vi "accel adjusted with gravity into ms2 (SubVI).vi"(10 "Array in":dbl[](array[numeric]), 11 "Array out":dbl[](array[numeric])) -> (3 "Array out":dbl[](array[numeric]))   [LabVIEW 2011]
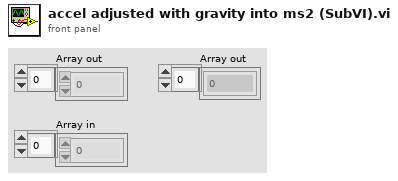
[diagram p1: front panel]
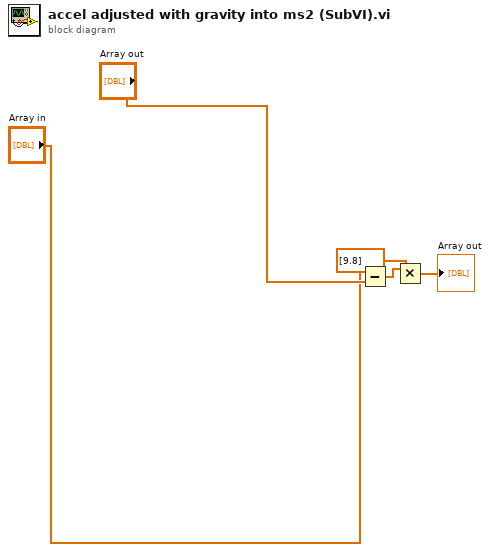
[diagram p0: block diagram]
diagram:
  n1 = Subtract(x="Array in", y="Array out") -> (x-y=w3:dbl[])
  n2 = Multiply(x=w3, y=dbl[] [9.8]) -> (x*y=→"Array out":dbl[])
